vi "Read Pre AIV Values.vi"(8 "error in":errorcluster, 11 "DAC HeatFlow Load dU in":refnum<class "DAC HeatFlow Load dU.lvclass">) -> (0 "error out":errorcluster, 3 "DAC HeatFlow Load dU out":refnum<class "DAC HeatFlow Load dU.lvclass">)   [LabVIEW 2019, in "DAC.lvlib" / "DAC HeatFlow Load dU.lvclass"]
uses:
  DAC HeatFlow Load dU.lvclass
  Results/Heat Flow Results/Heat Flow Results.lvclass
  Results/Results Method.ctl
  Results/Results.lvlib
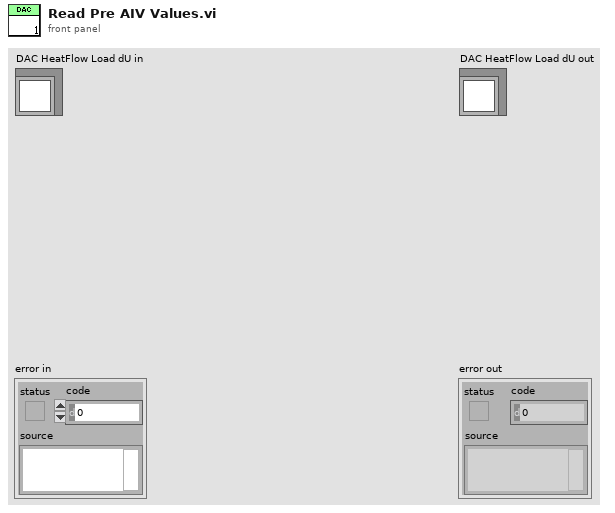
[diagram p1: front panel]
types:
  T1 = typedef "Results.lvlib/Results Method.ctl" = enum16{"Get", "Set"}
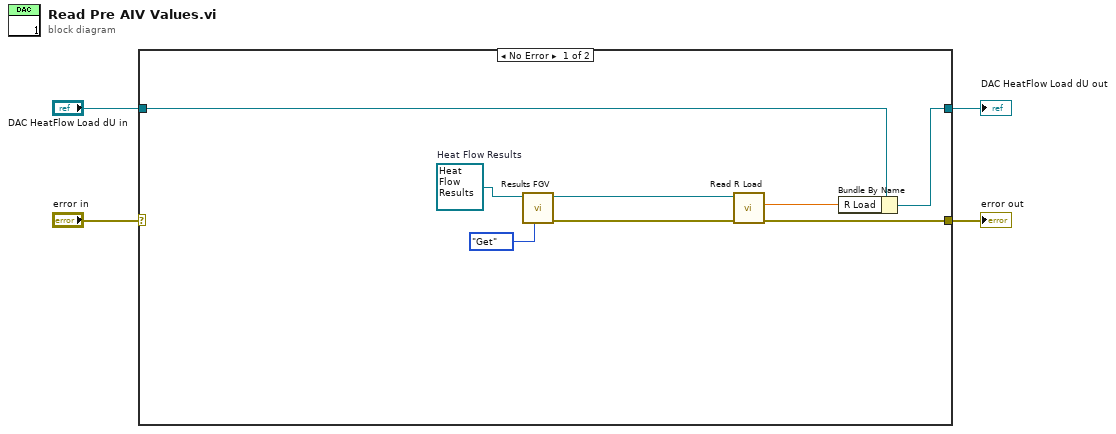
[diagram p0: block diagram]
diagram:
  n1 = case shown="No Error" "error in" {
    selector: "error in" -> [_ w14]
    tunnel: [w5 w14] -> w3
    tunnel: [w12 w13] -> w1
    tunnel: "DAC HeatFlow Load dU in" -> [w11 w13]
    frame No Error {
      w10 = refnum<class "Heat Flow Results.lvclass"> refnum  # Heat Flow Results
      n2 = call-dynamic "Results FGV.vi"("Method"=Results_Method."Get", "Results in"=w10) -> ("error out"=w6:errorcluster, "Results out"=w8:refnum<class "Heat Flow Results.lvclass">)  [unwired: 8 in]
      n3 = call "Read R Load.vi"("error in (no error)"=w6, "Heat Flow Results in"=w8) -> ("error out"=w5:errorcluster, "R Load"=w7:dbl)  [unwired: 7 in, 1 out]
      n4 = Bundle By Name(cluster=w11, "R Load"=w7) -> (w12:refnum<class "DAC HeatFlow Load dU.lvclass">)
    }
    frame Error {
    }
  }
  "error out" <- w3
  "DAC HeatFlow Load dU out" <- w1
